vi "Receive Message.vi"(8 "error in (no error)":errorcluster, 9 "timeout ms (25000)":i32, 10 "bytes to read":i32, 11 "object in":refnum<class "Laser_Ethernet.lvclass">) -> (0 "error out":errorcluster, 2 "Data":string, 3 "object out":refnum<class "Laser_Ethernet.lvclass">)   [LabVIEW 2023, in "Laser_Ethernet.lvclass"]
uses:
  Laser_Ethernet.lvclass
  Laser_Ethernet.lvclass/Laser_Ethernet.ctl
panel:
  out "Checksum OK":bool
  out "Data Size":u32
  out "Execution Code":u16
  out "Answer":u16
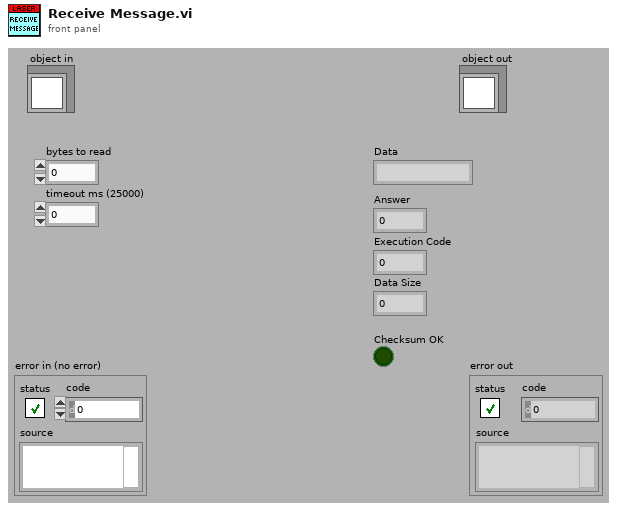
[diagram p1: front panel]
types:
  T1 = enum16{"big-endian, network order", "native, host order", "little-endian"}
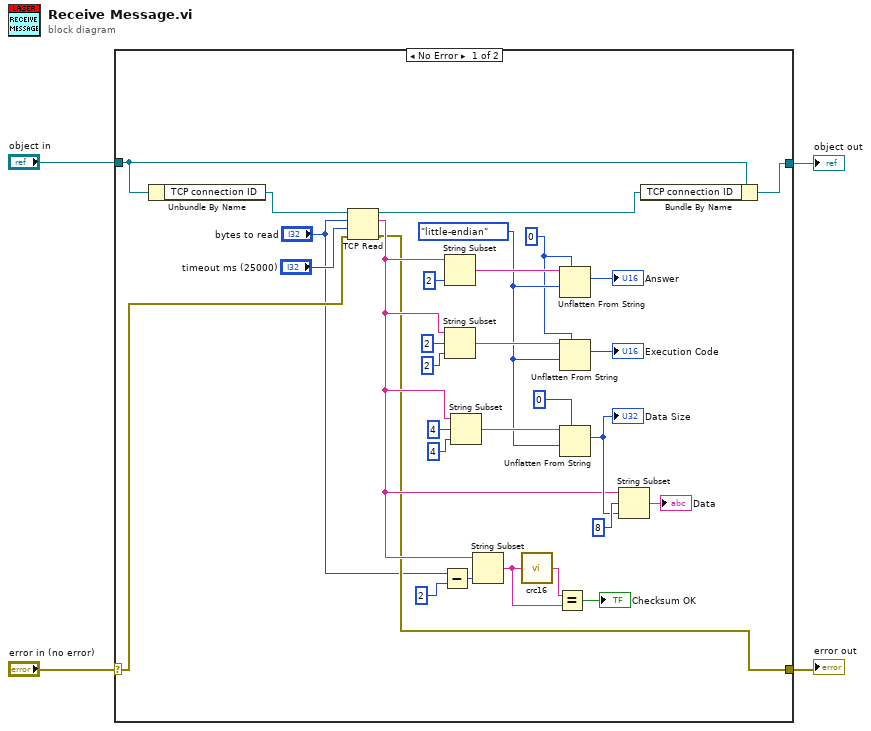
[diagram p0: block diagram]
diagram:
  n1 = case shown="No Error" "error in (no error)" {
    selector: "error in (no error)" -> [w12 w36]
    tunnel: [w11 w36] -> w3
    tunnel: [w6 w35] -> w1
    tunnel: "object in" -> [w7 w35]
    frame No Error {
      w23 = u16 0 ("offset (0)")
      w27 = T1."little-endian" ("byte order (0:big-endian, network order)")
      n2 = Unbundle By Name(w7) -> ("TCP connection ID"=w13:refnum<k5>)
      n3 = TCP Read(connection ID=w13, bytes to read="bytes to read", error in (no error)=w12, 9:"timeout ms (25000)") -> (connection ID out=w5:refnum<k5>, data out=w14:string, error out=w11:errorcluster)  [unwired: 1 in]
      n4 = Subtract(x="bytes to read", y=2) -> (x-y=w16:i32)
      n5 = String Subset(string=w14, length (rest)=2 ("length (rest)")) -> (substring=w32:string)  [unwired: 1 in]
      n6 = String Subset(string=w14, offset (0)=2, length (rest)=2 ("length (rest)")) -> (substring=w31:string)
      n7 = String Subset(string=w14, offset (0)=4, length (rest)=4 ("length (rest)")) -> (substring=w28:string)
      n8 = String Subset(string=w14, length (rest)=w16) -> (substring=w10:string)  [unwired: 1 in]
      n9 = call "crc16.vi"("Message"=w10) -> ("crc 16"=w9:string)
      n10 = Equal?(x=w9, y=w10) -> (x = y?=→"Checksum OK":bool)
      n11 = Unflatten From String(type=w23, binary string=w32, byte order (0:big-endian, network order)=w27) -> (value=→"Answer":u16)  [unwired: 2 in, 2 out]
      n12 = Unflatten From String(type=w23, binary string=w31, byte order (0:big-endian, network order)=w27) -> (value=→"Execution Code":u16)  [unwired: 2 in, 2 out]
      n13 = Unflatten From String(type=u32 0 ("offset (0)"), binary string=w28, byte order (0:big-endian, network order)=w27) -> (value=w21:u32)  [unwired: 2 in, 2 out]
      "Data Size" <- w21
      n14 = String Subset(string=w14, offset (0)=8, length (rest)=w21) -> (substring=→"Data":string)
      n15 = Bundle By Name(cluster=w7, "TCP connection ID"=w5) -> (w6:refnum<class "Laser_Ethernet.lvclass">)
    }
    frame Error {
    }
  }
  "error out" <- w3
  "object out" <- w1
